vi "UpdateGainOnChange.vi"(8 "error in":errorcluster, 10 "Gain":string(combo)="0", 11 "VISA resource name in":refnum<visa-resource-name>) -> (0 "error out":errorcluster, 3 "VISA resource name out":refnum<visa-resource-name>)   [LabVIEW 2011]
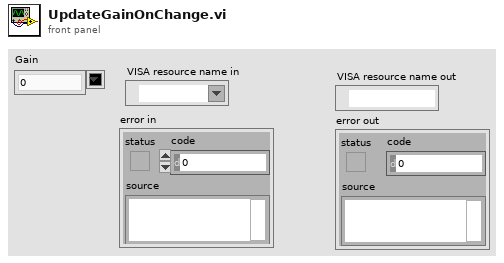
[diagram p1: front panel]
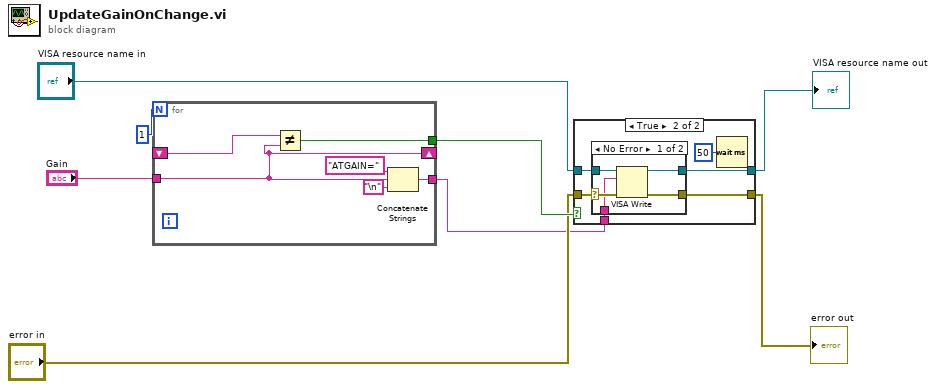
[diagram p0: block diagram]
diagram:
  n1 = for {
    N: 1 -> [_]
    shift-right: [w10] -> _
    shift-left: _ -> [w11]
    tunnel: [w9] -> w6
    tunnel: [w12] -> w3
    tunnel: "Gain" -> [w10]
    n2 = Not Equal?(x=w11, y=w10) -> (x != y?=w9:bool)
    n3 = Concatenate Strings("ATGAIN=", w10, "\n") -> (w12:string)
  }
  n4 = case shown="True" w6 {
    tunnel: [w16 w22] -> w2
    tunnel: [w15 w21] -> w1
    tunnel: "VISA resource name in" -> [w16 w20]
    tunnel: "error in" -> [w15 w19]
    tunnel: w3 -> [_ w18]
    frame False {
    }
    frame True {
      n5 = case shown="No Error" w19 {
        selector: w19 -> [w24 w29]
        tunnel: [w27 w28] -> w22
        tunnel: [w26 w29] -> w21
        tunnel: w20 -> [w25 w28]
        tunnel: w18 -> [w23 _]
        frame No Error {
          n6 = VISA Write(VISA resource name=w25, write buffer=w23, error in (no error)=w24) -> (VISA resource name out=w27:refnum<visa-resource-name>, error out=w26:errorcluster)  [unwired: 1 out]
        }
        frame Error {
        }
      }
      n7 = Wait (ms)(milliseconds to wait=u32 50) -> ()  [unwired: 1 out]
    }
  }
  "VISA resource name out" <- w2
  "error out" <- w1
